vi "NM GlobalTest.vi"() -> ()   [LabVIEW 2010] (continued)
                      n358 = call "NITrapBlankChan.vi"("error in (no error)"=w832) -> ("error out"=w829:errorcluster)  [unwired: 9 in, 1 out]
                      n359 = call-poly <vilib>:"DAQmx Create Virtual Channel.vi"("task in"=w831, "high ticks"="high ticks", "low ticks"="low ticks", "counter"="DAQmx", "source of ticks"="source of ticks", "error in"=w829, "idle state"="idle state", "initial delay"="initial delay") -> ("task out"=w830:refnum<k21>, "error out"=w828:errorcluster)  [unwired: 6 in]
                      n360 = call "NITrapBlankChan.vi"("error in (no error)"=w828) -> ("error out"=w827:errorcluster)  [unwired: 9 in, 1 out]
                      n361 = call-poly <vilib>:"DAQmx Create Virtual Channel.vi"("task in"=w830, "high ticks"="high ticks", "low ticks"="low ticks", "counter"="DAQmx", "source of ticks"="source of ticks", "error in"=w827, "idle state"="idle state", "initial delay"="initial delay") -> ("task out"=w820:refnum<k21>, "error out"=w826:errorcluster)  [unwired: 6 in]
                      n362 = call "NITrapBlankChan.vi"("error in (no error)"=w826) -> ("message"=w818:string, "error out"=w819:errorcluster)  [unwired: 9 in]
                    }
                  }
                }
              }
            }
            frame "Composite In" {
              n363 = stacked-sequence {
                seq-local: [w846 _ _ _ _ _] -> [_ w867 _ _ _ _]
                seq-local: [w845 _ _ _ _ _] -> [_ w866 _ _ _ _]
                seq-local: [_ w865 _ _ _ _] -> [_ _ w881 _ _ _]
                seq-local: [_ w864 _ _ _ _] -> [_ _ w878 _ _ _]
                seq-local: [_ _ w880 _ _ _] -> [_ _ _ w908 _ _]
                seq-local: [_ _ w879 _ _ _] -> [_ _ _ w907 _ _]
                seq-local: [_ _ _ w906 _ _] -> [_ _ _ _ w916 _]
                seq-local: [_ _ _ w905 _ _] -> [_ _ _ _ w918 _]
                seq-local: [_ _ _ _ w916 _] -> [_ _ _ _ _ w927]
                seq-local: [_ _ _ _ w922 _] -> [_ _ _ _ _ w926]
                seq-local: ["ULx" _ _ _ _ _] -> [_ w857 _ _ _ _]
                seq-local: [_ w856 _ _ _ _] -> [_ _ w876 _ _ _]
                seq-local: [_ _ w875 _ _ _] -> [_ _ _ w893 _ _]
                seq-local: [_ _ _ w891 _ _] -> [_ _ _ _ w921 _]
                seq-local: [_ _ _ _ w919 _] -> [_ _ _ _ _ w924]
                tunnel: [_ _ _ _ _ w928] -> w837
                tunnel: [_ _ _ _ _ w929] -> w836
                tunnel: [_ _ _ _ _ w930] -> w835
                tunnel: [_ _ _ _ _ w923] -> w833
                frame #0 {
                  # "Composite Analog Input"
                  n364 = call-poly <vilib>:"ULx Create Virtual Channel.vi"("maximum value"="max", "minimum value"="min", "physical channels"="ULx") -> ("task out"=w855:refnum<k24>, "error out"=w853:errorcluster)  [unwired: 11 in]
                  n365 = call "TrapBlankChan.vi"("error in (no error)"=w853) -> ("error out"=w852:errorcluster)  [unwired: 9 in, 1 out]
                  n366 = call-poly <vilib>:"ULx Create Virtual Channel.vi"("task in"=w855, "maximum value"="max 9", "minimum value"="min 9", "physical channels"="physical channels 17", "error in"=w852) -> ("task out"=w854:refnum<k24>, "error out"=w851:errorcluster)  [unwired: 9 in]
                  n367 = call "TrapBlankChan.vi"("error in (no error)"=w851) -> ("error out"=w850:errorcluster)  [unwired: 9 in, 1 out]
                  n368 = call-poly <vilib>:"ULx Create Virtual Channel.vi"("task in"=w854, "maximum value"="max 12", "minimum value"="min 12", "physical channels"="physical channels 18", "error in"=w850) -> ("task out"=w846:refnum<k24>, "error out"=w849:errorcluster)  [unwired: 9 in]
                  n369 = call "TrapBlankChan.vi"("error in (no error)"=w849) -> ("error out"=w845:errorcluster)  [unwired: 9 in, 1 out]
                }
                frame #1 {
                  # "Composite Temperature Input"
                  n370 = call "StringJoiner.vi"("string 2"="ULx", "string 1"=w857) -> ("concatenated string"=w856:string)
                  n371 = call-poly <vilib>:"ULx Create Virtual Channel.vi"("task in"=w867, "physical channels"="ULx", "units"="units", "error in"=w866) -> ("task out"=w874:refnum<k24>, "error out"=w872:errorcluster)  [unwired: 10 in]
                  n372 = call "TrapBlankChan.vi"("error in (no error)"=w872) -> ("error out"=w871:errorcluster)  [unwired: 9 in, 1 out]
                  n373 = call-poly <vilib>:"ULx Create Virtual Channel.vi"("task in"=w874, "physical channels"="physical channels 20", "units"="units 7", "error in"=w871) -> ("task out"=w873:refnum<k24>, "error out"=w870:errorcluster)  [unwired: 10 in]
                  n374 = call "TrapBlankChan.vi"("error in (no error)"=w870) -> ("error out"=w869:errorcluster)  [unwired: 9 in, 1 out]
                  n375 = call-poly <vilib>:"ULx Create Virtual Channel.vi"("task in"=w873, "physical channels"="physical channels 21", "units"="units 12", "error in"=w869) -> ("task out"=w865:refnum<k24>, "error out"=w868:errorcluster)  [unwired: 10 in]
                  n376 = call "TrapBlankChan.vi"("error in (no error)"=w868) -> ("error out"=w864:errorcluster)  [unwired: 9 in, 1 out]
                }
                frame #2 {
                  # "Composite Digital Input"
                  n377 = call "StringJoiner.vi"("string 2"="ULx", "string 1"=w876) -> ("concatenated string"=w875:string)
                  n378 = call-poly <vilib>:"ULx Create Virtual Channel.vi"("task in"=w881, "ports"="ULx", "error in"=w878) -> ("task out"=w890:refnum<k24>, "error out"=w888:errorcluster)  [unwired: 11 in]
                  n379 = call "TrapBlankChan.vi"("error in (no error)"=w888) -> ("error out"=w887:errorcluster)  [unwired: 9 in, 1 out]
                  n380 = call-poly <vilib>:"ULx Create Virtual Channel.vi"("task in"=w890, "ports"="ports 2", "error in"=w887) -> ("task out"=w889:refnum<k24>, "error out"=w886:errorcluster)  [unwired: 11 in]
                  n381 = call "TrapBlankChan.vi"("error in (no error)"=w886) -> ("error out"=w885:errorcluster)  [unwired: 9 in, 1 out]
                  n382 = call-poly <vilib>:"ULx Create Virtual Channel.vi"("task in"=w889, "ports"="ports 3", "error in"=w885) -> ("task out"=w880:refnum<k24>, "error out"=w884:errorcluster)  [unwired: 11 in]
                  n383 = call "TrapBlankChan.vi"("error in (no error)"=w884) -> ("error out"=w879:errorcluster)  [unwired: 9 in, 1 out]
                }
                frame #3 {
                  # "Composite Counter Edge Input"
                  n384 = call "StringJoiner.vi"("string 2"="ULx", "string 1"=w893) -> ("concatenated string"=w891:string)
                  n385 = call-poly <vilib>:"ULx Create Virtual Channel.vi"("task in"=w908, "initial count"="initial count", "count direction"="direction", "edge"="edge", "counters"="ULx", "error in"=w907) -> ("task out"=w915:refnum<k24>, "error out"=w913:errorcluster)  [unwired: 8 in]
                  n386 = call "TrapBlankChan.vi"("error in (no error)"=w913) -> ("error out"=w912:errorcluster)  [unwired: 9 in, 1 out]
                  n387 = call-poly <vilib>:"ULx Create Virtual Channel.vi"("task in"=w915, "initial count"="initial count 5", "count direction"="direction 5", "edge"="edge 5", "counters"="counters 22", "error in"=w912) -> ("task out"=w914:refnum<k24>, "error out"=w911:errorcluster)  [unwired: 8 in]
                  n388 = call "TrapBlankChan.vi"("error in (no error)"=w911) -> ("error out"=w910:errorcluster)  [unwired: 9 in, 1 out]
                  n389 = call-poly <vilib>:"ULx Create Virtual Channel.vi"("task in"=w914, "initial count"="initial count 6", "count direction"="direction 6", "edge"="edge 6", "counters"="counters 23", "error in"=w910) -> ("task out"=w906:refnum<k24>, "error out"=w909:errorcluster)  [unwired: 8 in]
                  n390 = call "TrapBlankChan.vi"("error in (no error)"=w909) -> ("error out"=w905:errorcluster)  [unwired: 9 in, 1 out]
                }
                frame #4 {
                  # "Composite Encoder Input"
                  n391 = call "StringJoiner.vi"("string 2"="ULx", "string 1"=w921) -> ("concatenated string"=w919:string)
                  n392 = call "TrapBlankChan.vi"("error in (no error)"=w918) -> ("error out"=w917:errorcluster)  [unwired: 9 in, 1 out]
                  n393 = call "TrapBlankChan.vi"("error in (no error)"=w917) -> ("error out"=w922:errorcluster)  [unwired: 9 in, 1 out]
                }
                frame #5 {
                  n394 = call "StringJoiner.vi"("string 2"="ULx", "string 1"=w924) -> ("concatenated string"=w923:string)
                  n395 = call-poly <vilib>:"ULx Create Virtual Channel.vi"("task in"=w927, "maximum value"="max", "minimum value"="min", "physical channels"="ULx", "error in"=w926) -> ("task out"=w945:refnum<k24>, "error out"=w943:errorcluster)  [unwired: 9 in]
                  n396 = call "TrapBlankChan.vi"("error in (no error)"=w943) -> ("error out"=w942:errorcluster)  [unwired: 9 in, 1 out]
                  n397 = call-poly <vilib>:"ULx Create Virtual Channel.vi"("task in"=w945, "maximum value"="max 15", "minimum value"="min 15", "physical channels"="physical channels 29", "error in"=w942) -> ("task out"=w944:refnum<k24>, "error out"=w941:errorcluster)  [unwired: 9 in]
                  n398 = call "TrapBlankChan.vi"("error in (no error)"=w941) -> ("error out"=w940:errorcluster)  [unwired: 9 in, 1 out]
                  n399 = call-poly <vilib>:"ULx Create Virtual Channel.vi"("task in"=w944, "maximum value"="max 18", "minimum value"="min 18", "physical channels"="physical channels 30", "error in"=w940) -> ("task out"=w930:refnum<k24>, "error out"=w939:errorcluster)  [unwired: 9 in]
                  n400 = call "TrapBlankChan.vi"("error in (no error)"=w939) -> ("message"=w928:string, "error out"=w929:errorcluster)  [unwired: 9 in]
                }
              }
            }
            frame "Composite Out" {
              n401 = stacked-sequence {
                seq-local: [w961 _ _] -> [_ w977 _]
                seq-local: [w960 _ _] -> [_ w976 _]
                seq-local: [_ w975 _] -> [_ _ w992]
                seq-local: [_ w974 _] -> [_ _ w991]
                seq-local: ["ULx" _ _] -> [_ w971 _]
                seq-local: [_ w969 _] -> [_ _ w987]
                tunnel: [_ _ w990] -> w948
                tunnel: [_ _ w989] -> w950
                tunnel: [_ _ w988] -> w949
                tunnel: [_ _ w985] -> w946
                frame #0 {
                  # "Composite Analog Output"
                  n402 = call-poly <vilib>:"ULx Create Virtual Channel.vi"("maximum value"="max", "minimum value"="min", "physical channels"="ULx") -> ("task out"=w968:refnum<k24>, "error out"=w966:errorcluster)  [unwired: 11 in]
                  n403 = call "TrapBlankChan.vi"("error in (no error)"=w966) -> ("error out"=w965:errorcluster)  [unwired: 9 in, 1 out]
                  n404 = call-poly <vilib>:"ULx Create Virtual Channel.vi"("task in"=w968, "maximum value"="max 13", "minimum value"="min 13", "physical channels"="physical channels 23", "error in"=w965) -> ("task out"=w967:refnum<k24>, "error out"=w964:errorcluster)  [unwired: 9 in]
                  n405 = call "TrapBlankChan.vi"("error in (no error)"=w964) -> ("error out"=w963:errorcluster)  [unwired: 9 in, 1 out]
                  n406 = call-poly <vilib>:"ULx Create Virtual Channel.vi"("task in"=w967, "maximum value"="max 14", "minimum value"="min 14", "physical channels"="physical channels 24", "error in"=w963) -> ("task out"=w961:refnum<k24>, "error out"=w962:errorcluster)  [unwired: 9 in]
                  n407 = call "TrapBlankChan.vi"("error in (no error)"=w962) -> ("error out"=w960:errorcluster)  [unwired: 9 in, 1 out]
                }
                frame #1 {
                  # "Composite Digital Output"
                  n408 = call "StringJoiner.vi"("string 2"="ULx", "string 1"=w971) -> ("concatenated string"=w969:string)
                  n409 = call-poly <vilib>:"ULx Create Virtual Channel.vi"("task in"=w977, "ports"="ULx", "error in"=w976) -> ("task out"=w984:refnum<k24>, "error out"=w982:errorcluster)  [unwired: 11 in]
                  n410 = call "TrapBlankChan.vi"("error in (no error)"=w982) -> ("error out"=w981:errorcluster)  [unwired: 9 in, 1 out]
                  n411 = call-poly <vilib>:"ULx Create Virtual Channel.vi"("task in"=w984, "ports"="ports 5", "error in"=w981) -> ("task out"=w983:refnum<k24>, "error out"=w980:errorcluster)  [unwired: 11 in]
                  n412 = call "TrapBlankChan.vi"("error in (no error)"=w980) -> ("error out"=w979:errorcluster)  [unwired: 9 in, 1 out]
                  n413 = call-poly <vilib>:"ULx Create Virtual Channel.vi"("task in"=w983, "ports"="ports 6", "error in"=w979) -> ("task out"=w975:refnum<k24>, "error out"=w978:errorcluster)  [unwired: 11 in]
                  n414 = call "TrapBlankChan.vi"("error in (no error)"=w978) -> ("error out"=w974:errorcluster)  [unwired: 9 in, 1 out]
                }
                frame #2 {
                  # "Repeat Composite Analog Output"
                  n415 = call "StringJoiner.vi"("string 2"="ULx", "string 1"=w987) -> ("concatenated string"=w985:string)
                  n416 = call-poly <vilib>:"ULx Create Virtual Channel.vi"("task in"=w992, "maximum value"="max", "minimum value"="min", "physical channels"="ULx", "error in"=w991) -> ("task out"=w1007:refnum<k24>, "error out"=w1005:errorcluster)  [unwired: 9 in]
                  n417 = call "TrapBlankChan.vi"("error in (no error)"=w1005) -> ("error out"=w1004:errorcluster)  [unwired: 9 in, 1 out]
                  n418 = call-poly <vilib>:"ULx Create Virtual Channel.vi"("task in"=w1007, "maximum value"="max 16", "minimum value"="min 16", "physical channels"="physical channels 26", "error in"=w1004) -> ("task out"=w1006:refnum<k24>, "error out"=w1003:errorcluster)  [unwired: 9 in]
                  n419 = call "TrapBlankChan.vi"("error in (no error)"=w1003) -> ("error out"=w1002:errorcluster)  [unwired: 9 in, 1 out]
                  n420 = call-poly <vilib>:"ULx Create Virtual Channel.vi"("task in"=w1006, "maximum value"="max 17", "minimum value"="min 17", "physical channels"="physical channels 27", "error in"=w1002) -> ("task out"=w990:refnum<k24>, "error out"=w1001:errorcluster)  [unwired: 9 in]
                  n421 = call "TrapBlankChan.vi"("error in (no error)"=w1001) -> ("message"=w988:string, "error out"=w989:errorcluster)  [unwired: 9 in]
                }
              }
            }
          }
          n422 = local write "Active Channels"(w143) -> ()
          n423 = for {
            N: 5 -> [_]
            tunnel: w146 -> [w1009]
            tunnel: [FALSE] -> w145
            n424 = Wait Until Next ms Multiple(millisecond multiple=w1009) -> ()  [unwired: 1 out]
            "CreateChans" <- TRUE
          }
          n425 = case shown="No Error" w149 {
            selector: w149 -> [w1011 w1013]
            tunnel: [w1011 w1013] -> w152
            tunnel: w148 -> [_ w1012]
            frame No Error {
            }
            frame Error {
              "message 2" <- w1012
            }
          }
          n426 = local write "CreateChans"(w145) -> ()
        }
        frame 3 {
          # "Channel Info"
          n427 = Not Equal?(x="", y="Active Channels") -> (x != y?=w1014:bool)
          n428 = case shown="True" w1014 {
            tunnel: w1024 -> [w1033 w1041]
            tunnel: w1023 -> [w1032 w1040]
            tunnel: w1022 -> [w1031 w1039]
            tunnel: [w1033 w1038] -> w1021
            tunnel: [w1032 w1037] -> w1020
            tunnel: [w1031 w1036] -> w1019
            tunnel: w1018 -> [_ w1035]
            tunnel: "Active Channels" -> [_ w1034]
            frame False {
            }
            frame True {
              n429 = case shown="\"ULx\", Default" w1035 {
                tunnel: w1039 -> [w1045 w1053]
                tunnel: w1041 -> [w1047 w1052]
                tunnel: [w1047 w1051] -> w1038
                tunnel: [w1044 w1050] -> w1036
                tunnel: w1040 -> [w1043 w1049]
                tunnel: [w1042 w1049] -> w1037
                tunnel: w1034 -> [w1046 w1048]
                frame "ULx", Default {
                  n430 = call "SetActiveChans.vi"("error in (no error)"=w1045, "ActiveChannels"=w1046, "task in"=w1043) -> ("error out"=w1044:errorcluster, "task out"=w1042:refnum<k24>)
                }
                frame "DAQmx" {
                  n431 = property class="DAQmx Channel"(reference=w1052, error in=w1053, "ActiveChans"=w1048) -> (reference out=w1051:refnum<k21>, error out=w1050:errorcluster)
                }
              }
            }
          }
          n432 = call "DAQmxTaskInfo.vi"("task in"=w1021) -> ("ChanType"=→"ChanType":i32, "Name"=→"Name":refnum<k21>)
          n433 = call "ULxTaskInfo.vi"("task in"=w1020) -> ("NumberOfChannels"=→"NumberOfChannels":u32, "Task"=→"Task":i32, "ToString"=→"ToString":string)
          n434 = local read "SelLib"() -> (w1025:enum32{"ULx", "DAQmx"})
          n435 = case shown="\"ULx\", Default" w1025 {
            tunnel: w1021 -> [_ w1058]
            tunnel: w1020 -> [w1056 _]
            tunnel: [w1054 w1057] -> w1026
            frame "ULx", Default {
              n436 = call "ULxTaskInfo.vi"("task in"=w1056) -> ("Task"=w1055:i32)  [unwired: 2 out]
              n437 = Number To Hexadecimal String(2:w1055) -> (0:w1054:string)  [unwired: 1 in]
            }
            frame "DAQmx" {
              n438 = call "DAQmxTaskInfo.vi"("task in"=w1058) -> ("Name"=w1057:refnum<k21>)  [unwired: 1 out]
            }
          }
          "String" <- w1026
        }
        frame 4 {
          # "TIMING"
          n439 = for {
            N: 5 -> [_]
            tunnel: w1061 -> [w1073]
            tunnel: [FALSE] -> w1060
            n440 = Wait Until Next ms Multiple(millisecond multiple=w1073) -> ()  [unwired: 1 out]
            "Timing" <- TRUE
          }
          n441 = local write "Timing"(w1060) -> ()
          n442 = case shown="\"Clock\", Default" "Tab Control" {
            tunnel: w1067 -> [w1081 w1107 w1128]
            tunnel: w1066 -> [w1080 w1106 w1127]
            tunnel: [w1079 w1105 w1126] -> w1064
            tunnel: [w1078 w1104 w1125] -> w1063
            tunnel: w1069 -> [w1077 w1103 w1124]
            tunnel: w1068 -> [w1076 w1102 w1123]
            tunnel: [w1075 w1101 w1122] -> w1065
            frame "Clock", Default {
              n443 = case shown="\"DAQmx\"" w1077 {
                tunnel: w1081 -> [w1090 w1091]
                tunnel: w1080 -> [w1089 w1100]
                tunnel: [w1088 w1091] -> w1079
                tunnel: [w1087 w1099] -> w1078
                tunnel: w1076 -> [w1082 w1098]
                tunnel: [w1082 w1097] -> w1075
                frame "ULx", Default {
                  n444 = call-poly <vilib>:"ULx Timing.vi"("task in"=w1090, "sample mode"="sample mode", "samples per channel"="samples per", "rate"="rate", "clock source"="clock source", "error in"=w1089) -> ("task out"=w1088:refnum<k24>, "error out"=w1087:errorcluster)  [unwired: 8 in]
                }
                frame "DAQmx" {
                  n445 = call-poly <vilib>:"DAQmx Timing.vi"("task/channels in"=w1098, "sample mode"="sample mode", "samples per channel"="samples per", "rate"="mxRate", "source"="source", "active edge"="active edge", "error in"=w1100) -> ("task out"=w1097:refnum<k21>, "error out"=w1099:errorcluster)  [unwired: 7 in]
                }
              }
            }
            frame "Waveform" {
              n446 = case shown="\"ULx\", Default" w1103 {
                tunnel: w1107 -> [w1114 w1115]
                tunnel: w1106 -> [w1113 w1121]
                tunnel: [w1112 w1115] -> w1105
                tunnel: [w1111 w1120] -> w1104
                tunnel: w1102 -> [w1108 w1119]
                tunnel: [w1108 w1118] -> w1101
                frame "ULx", Default {
                  n447 = call-poly <vilib>:"ULx Timing.vi"("task in"=w1114, "sample mode"="sample mode 3", "waveform"="waveform", "error in"=w1113) -> ("task out"=w1112:refnum<k24>, "error out"=w1111:errorcluster)  [unwired: 10 in]
                }
                frame "DAQmx" {
                  n448 = call-poly <vilib>:"DAQmx Timing.vi"("task/channels in"=w1119, "sample mode"="sample mode 2", "waveform"="waveform 2", "error in"=w1121) -> ("task out"=w1118:refnum<k21>, "error out"=w1120:errorcluster)  [unwired: 10 in]
                }
              }
            }
            frame "Implicit" {
              n449 = case shown="\"ULx\", Default" w1124 {
                tunnel: w1128 -> [w1135 w1136]
                tunnel: w1127 -> [w1134 w1142]
                tunnel: [w1133 w1136] -> w1126
                tunnel: [w1132 w1141] -> w1125
                tunnel: w1123 -> [w1131 w1140]
                tunnel: [w1131 w1139] -> w1122
                frame "ULx", Default {
                  n450 = call-poly <vilib>:"ULx Timing.vi"("task in"=w1135, "sample mode"="sample mode", "samples per channel"="samples per channel", "error in"=w1134) -> ("task out"=w1133:refnum<k24>, "error out"=w1132:errorcluster)  [unwired: 10 in]
                }
                frame "DAQmx" {
                  n451 = call-poly <vilib>:"DAQmx Timing.vi"("task/channels in"=w1140, "sample mode"="sample mode", "samples per channel"="samples per channel", "error in"=w1142) -> ("task out"=w1139:refnum<k21>, "error out"=w1141:errorcluster)  [unwired: 10 in]
                }
              }
            }
          }
          n452 = case shown="True" "Once" {
            frame False {
            }
            frame True {
              n453 = local write "Timing"(FALSE ("Timing")) -> ()
            }
          }
        }
        frame 5 {
          # "TRIGGERING"
          n454 = for {
            N: 5 -> [_]
            tunnel: w1145 -> [w1161]
            tunnel: [FALSE] -> w1144
            n455 = Wait Until Next ms Multiple(millisecond multiple=w1161) -> ()  [unwired: 1 out]
            "Trigger" <- TRUE
          }
          n456 = case shown="\"Basic\", Default" "TrigType" {
            tunnel: [w1169 w1241 w1292 w1348] -> w1156
            tunnel: [w1170 w1240 w1293 w1349] -> w1157
            tunnel: "BasicType" -> [w1168 _ _ _]
            tunnel: "GatedType" -> [_ w1239 _ _]
            tunnel: "StartType" -> [_ _ w1294 _]
            tunnel: "StopType" -> [_ _ _ w1350]
            tunnel: [w1167 w1238 w1290 w1344] -> w1158
            tunnel: w1150 -> [w1165 w1236 w1289 w1347]
            tunnel: w1149 -> [w1164 w1235 w1288 w1346]
            tunnel: w1148 -> [w1166 w1237 w1291 w1345]
            tunnel: w1147 -> [w1163 w1234 _ _]
            frame "Basic", Default {
              n457 = case shown="\"DPtrn\"" w1168 {
                tunnel: [w1177 w1194 w1213 w1219 w1231] -> w1170
                tunnel: [w1176 w1193 w1214 w1218 w1232] -> w1169
                tunnel: [w1175 w1192 w1215 w1225 w1233] -> w1167
                tunnel: w1166 -> [w1174 w1191 w1215 w1225 w1233]
                tunnel: w1165 -> [w1173 w1190 w1209 w1217 w1227]
                tunnel: w1164 -> [w1172 w1189 w1210 w1216 w1226]
                tunnel: w1163 -> [w1171 w1188 _ _ _]
                frame "None", Default {
                  n458 = case shown="\"ULx\", Default" w1171 {
                    tunnel: [w1181 w1184] -> w1177
                    tunnel: [w1180 w1187] -> w1176
                    tunnel: [w1182 w1186] -> w1175
                    tunnel: w1174 -> [w1182 w1185]
                    tunnel: w1173 -> [w1179 w1184]
                    tunnel: w1172 -> [w1178 w1183]
                    frame "ULx", Default {
                      n459 = call-poly <vilib>:"ULx Trigger.vi"("task in"=w1179, "error in"=w1178) -> ("task out"=w1181:refnum<k24>, "error out"=w1180:errorcluster)  [unwired: 16 in]
                    }
                    frame "DAQmx" {
                      n460 = call-poly <vilib>:"DAQmx Trigger.vi"("task/channels in"=w1185, "error in"=w1183) -> ("task out"=w1186:refnum<k21>, "error out"=w1187:errorcluster)  [unwired: 12 in]
                    }
                  }
                }
                frame "DEdge" {
                  n461 = case shown="\"ULx\", Default" w1188 {
                    tunnel: [w1198 w1203] -> w1194
                    tunnel: [w1199 w1208] -> w1193
                    tunnel: [w1201 w1207] -> w1192
                    tunnel: w1191 -> [w1201 w1204]
                    tunnel: w1190 -> [w1195 w1203]
                    tunnel: w1189 -> [w1196 w1202]
                    frame "ULx", Default {
                      n462 = call-poly <vilib>:"ULx Trigger.vi"("task in"=w1195, "edge"="ULx edge", "error in"=w1196, "pretrigger samples per channel"="pretrigger samples per channel") -> ("task out"=w1198:refnum<k24>, "error out"=w1199:errorcluster)  [unwired: 14 in]
                    }
                    frame "DAQmx" {
                      n463 = call-poly <vilib>:"DAQmx Trigger.vi"("task/channels in"=w1204, "source"="DAQmx source", "edge"="DAQmx edge", "error in"=w1202) -> ("task out"=w1207:refnum<k21>, "error out"=w1208:errorcluster)  [unwired: 10 in]
                    }
                  }
                }
                frame "DLevel" {
                  n464 = call-poly <vilib>:"ULx Trigger.vi"("task in"=w1209, "level"="level", "error in"=w1210, "pretrigger samples per channel"="pretrigger samples per channel") -> ("task out"=w1213:refnum<k24>, "error out"=w1214:errorcluster)  [unwired: 14 in]
                }
                frame "DPtrn" {
                  n465 = call-poly <vilib>:"ULx Trigger.vi"("task in"=w1217, "trigger channel"="trig chan", "trigger sensitivity"="sensitivity", "pattern"="pattern", "mask"="mask", "error in"=w1216, "pretrigger samples per channel"="Pretrig Samps") -> ("task out"=w1219:refnum<k24>, "error out"=w1218:errorcluster)  [unwired: 11 in]
                }
                frame "AEdge" {
                  n466 = call-poly <vilib>:"ULx Trigger.vi"("task in"=w1227, "slope"="slope", "level"="level", "error in"=w1226, "pretrigger samples per channel"="pretrigger samples per channel") -> ("task out"=w1231:refnum<k24>, "error out"=w1232:errorcluster)  [unwired: 13 in]
                }
              }
            }
            frame "Gated" {
              n467 = case shown="\"None\", Default" w1239 {
                tunnel: [w1247 w1263 w1270 w1278 w1286] -> w1241
                tunnel: [w1248 w1262 w1269 w1277 w1285] -> w1240
                tunnel: [w1246 w1264 w1271 w1279 w1287] -> w1238
                tunnel: w1237 -> [w1245 w1264 w1271 w1279 w1287]
                tunnel: w1236 -> [w1244 w1259 w1265 w1272 w1280]
                tunnel: w1235 -> [w1243 w1260 w1266 w1273 w1281]
                tunnel: w1234 -> [w1242 _ _ _ _]
                frame "None", Default {
                  n468 = case shown="\"ULx\", Default" w1242 {
                    tunnel: [w1252 w1255] -> w1248
                    tunnel: [w1251 w1258] -> w1247
                    tunnel: [w1253 w1257] -> w1246
                    tunnel: w1245 -> [w1253 w1256]
                    tunnel: w1244 -> [w1249 w1255]
                    tunnel: w1243 -> [w1250 w1254]
                    frame "ULx", Default {
                      n469 = call-poly <vilib>:"ULx Trigger.vi"("task in"=w1249, "error in"=w1250) -> ("task out"=w1252:refnum<k24>, "error out"=w1251:errorcluster)  [unwired: 16 in]
                    }
                    frame "DAQmx" {
                      n470 = call-poly <vilib>:"DAQmx Trigger.vi"("task/channels in"=w1256, "error in"=w1254) -> ("task out"=w1257:refnum<k21>, "error out"=w1258:errorcluster)  [unwired: 12 in]
                    }
                  }
                }
                frame "DLevel" {
                  n471 = call-poly <vilib>:"ULx Trigger.vi"("task in"=w1259, "level"="Level 3", "error in"=w1260) -> ("task out"=w1262:refnum<k24>, "error out"=w1263:errorcluster)  [unwired: 15 in]
                }
                frame "ALevel" {
                  n472 = call-poly <vilib>:"ULx Trigger.vi"("task in"=w1265, "position"="position", "level"="level", "error in"=w1266) -> ("task out"=w1269:refnum<k24>, "error out"=w1270:errorcluster)  [unwired: 14 in]
                }
                frame "AWindow" {
                  n473 = call-poly <vilib>:"ULx Trigger.vi"("task in"=w1272, "When"="When", "window bottom"="bottom", "window top"="top", "error in"=w1273) -> ("task out"=w1277:refnum<k24>, "error out"=w1278:errorcluster)  [unwired: 13 in]
                }
                frame "AHyst" {
                  n474 = call-poly <vilib>:"ULx Trigger.vi"("task in"=w1280, "hysteresis"="hyst", "low threshold"="low", "high threshold"="high", "error in"=w1281) -> ("task out"=w1285:refnum<k24>, "error out"=w1286:errorcluster)  [unwired: 13 in]
                }
              }
            }
            frame "Start" {
              n475 = case shown="\"None\", Default" w1294 {
                tunnel: [w1298 w1303 w1311 w1321 w1331 w1341] -> w1293
                tunnel: [w1295 w1304 w1312 w1322 w1332 w1342] -> w1292
                tunnel: [w1299 w1305 w1313 w1323 w1333 w1343] -> w1290
                tunnel: w1291 -> [w1299 w1305 w1313 w1323 w1333 w1343]
                tunnel: w1289 -> [w1297 w1301 w1306 w1314 w1324 w1334]
                tunnel: w1288 -> [w1296 w1302 w1307 w1315 w1325 w1335]
                frame "None", Default {
                  n476 = call-poly <vilib>:"ULx Trigger.vi"("task in"=w1297, "error in"=w1296) -> ("task out"=w1298:refnum<k24>, "error out"=w1295:errorcluster)  [unwired: 16 in]
                }
                frame "ExtTTL" {
                  n477 = call-poly <vilib>:"ULx Trigger.vi"("task in"=w1301, "trigger sensitivity"="trigger sensitivity", "error in"=w1302) -> ("task out"=w1303:refnum<k24>, "error out"=w1304:errorcluster)  [unwired: 15 in]
                }
                frame "AHdwr" {
                  n478 = call-poly <vilib>:"ULx Trigger.vi"("task in"=w1306, "trigger sensitivity"="sensitivity", "level"="Level", "variance"="variance", "error in"=w1307) -> ("task out"=w1311:refnum<k24>, "error out"=w1312:errorcluster)  [unwired: 13 in]
                }
                frame "ASftwr" {
                  n479 = call-poly <vilib>:"ULx Trigger.vi"("task in"=w1314, "trigger channel"="trigger channel", "trigger sensitivity"="sensitivity", "level"="Level", "variance"="variance", "error in"=w1315, "pretrigger samples per channel"="pretrigger samples") -> ("task out"=w1321:refnum<k24>, "error out"=w1322:errorcluster)  [unwired: 11 in]
                }
                frame "DPtrn" {
                  n480 = call-poly <vilib>:"ULx Trigger.vi"("task in"=w1324, "trigger channel"="trigger channel", "trigger sensitivity"="trigger sensitivity", "pattern"="level", "variance"="variance", "error in"=w1325, "pretrigger samples per channel"="pretrigger samples") -> ("task out"=w1331:refnum<k24>, "error out"=w1332:errorcluster)  [unwired: 11 in]
                }
                frame "Ctr" {
                  n481 = call-poly <vilib>:"ULx Trigger.vi"("task in"=w1334, "trigger channel"="trigger channel", "trigger sensitivity"="trigger sensitivity", "count"="level", "variance"="variance", "error in"=w1335, "pretrigger samples per channel"="pretrigger samples") -> ("task out"=w1341:refnum<k24>, "error out"=w1342:errorcluster)  [unwired: 11 in]
                }
              }
            }
            frame "Stop" {
              n482 = case shown="\"None\", Default" w1350 {
                tunnel: [w1351 w1362 w1371 w1380] -> w1349
                tunnel: [w1353 w1363 w1372 w1381] -> w1348
                tunnel: w1347 -> [w1352 w1357 w1365 w1374]
                tunnel: w1346 -> [w1354 w1356 w1366 w1375]
                tunnel: w1345 -> [w1355 w1364 w1373 w1382]
                tunnel: [w1355 w1364 w1373 w1382] -> w1344
                frame "None", Default {
                  n483 = call-poly <vilib>:"ULx Trigger.vi"("task in"=w1352, "error in"=w1354) -> ("task out"=w1351:refnum<k24>, "error out"=w1353:errorcluster)  [unwired: 16 in]
                }
                frame "ASftwr" {
                  n484 = call-poly <vilib>:"ULx Trigger.vi"("task in"=w1357, "trigger channel"="trigger channel", "trigger sensitivity"="trigger sensitivity", "level"="level", "variance"="variance", "error in"=w1356) -> ("task out"=w1362:refnum<k24>, "error out"=w1363:errorcluster)  [unwired: 12 in]
                }
                frame "DPtrn" {
                  n485 = call-poly <vilib>:"ULx Trigger.vi"("task in"=w1365, "trigger channel"="trigger channel", "trigger sensitivity"="trigger sensitivity", "pattern"="level", "variance"="variance", "error in"=w1366) -> ("task out"=w1371:refnum<k24>, "error out"=w1372:errorcluster)  [unwired: 12 in]
                }
                frame "Ctr" {
                  n486 = call-poly <vilib>:"ULx Trigger.vi"("task in"=w1374, "trigger channel"="trigger channel", "trigger sensitivity"="trigger sensitivity", "count"="level", "variance"="variance", "error in"=w1375) -> ("task out"=w1380:refnum<k24>, "error out"=w1381:errorcluster)  [unwired: 12 in]
                }
              }
            }
          }
          n487 = local write "Trigger"(w1144) -> ()
          n488 = case shown="True" "Once" {
            frame False {
            }
            frame True {
              n489 = local write "Trig"(FALSE ("Trig")) -> ()
            }
          }
        }
        frame 6 {
          # "START"
          n490 = for {
            N: 5 -> [_]
            tunnel: w1391 -> [w1401]
            tunnel: w1390 -> [w1400]
            tunnel: [FALSE] -> w1389
            n491 = case shown="1" w1400 {
              tunnel: TRUE -> [w1402 w1403]
              frame 0, Default {
                "Start" <- w1402
              }
              frame 1 {
                "Start 2" <- w1403
              }
            }
            n492 = Wait Until Next ms Multiple(millisecond multiple=w1401) -> ()  [unwired: 1 out]
          }
          n493 = case shown="\"DAQmx\"" w1386 {
            tunnel: w1394 -> [w1408 w1409]
            tunnel: [w1407 w1409] -> w1384
            tunnel: [w1406 w1412] -> w1383
            tunnel: w1393 -> [w1405 w1413]
            tunnel: w1395 -> [w1404 w1411]
            tunnel: [w1404 w1410] -> w1385
            frame "ULx", Default {
              n494 = call <vilib>:"ULx Start Task.vi"("task in"=w1408, "error in"=w1405) -> ("task out"=w1407:refnum<k24>, "error out"=w1406:errorcluster)  [unwired: 12 in]
            }
            frame "DAQmx" {
              n495 = call <vilib>:"DAQmx Start Task.vi"("task/channels in"=w1411, "error in"=w1413) -> ("task out"=w1410:refnum<k21>, "error out"=w1412:errorcluster)  [unwired: 12 in]
            }
          }
          n496 = local write "Start"(w1389) -> ()
          n497 = local write "Start 2"(w1389) -> ()
          n498 = case shown="True" "Once" {
            frame False {
            }
            frame True {
              n499 = local write "Start"(FALSE ("Start")) -> ()
            }
          }
          n500 = case shown="True" "Once" {
            frame False {
            }
            frame True {
              n501 = local write "Start"(FALSE ("Start")) -> ()
            }
          }
        }
        frame 7 {
          # "WRITE"
          n502 = property on="samples" class="DigNum (strict)"("Maximum"="samps") -> ()  [unwired: 2 in, 2 out]
          n503 = call "Complicated Function Generator.vi"("frequency"="freq", "signal type"="sig type", "offset"="offset", "amplitude"="ampl", "samples"="samps", "bufsize"="samps", "Chans"="Chans") -> ("Wave out"=w1424:waveform(dbl), "WfmArray"=w1422:waveform(dbl)[], "DblArray"=w1423:dbl[][], "DBL Out"=w1419:dbl[])  [unwired: 3 in, 2 out]
          n504 = case shown="False" "Mod Array" {
            tunnel: "Chans" -> [_ w1443]
            tunnel: w1419 -> [w1437 w1442]
            tunnel: [w1437 w1438] -> w1418
            frame False {
            }
            frame True {
              n505 = call "Complicated Function Generator.vi"("frequency"="freq", "signal type"="signal type", "amplitude"="atude", "samples"="samples", "bufsize"="samples", "Chans"=w1443) -> ("DBL Out"=w1445:dbl[])  [unwired: 4 in, 5 out]
              n506 = Replace Array Subset(array=w1442, new element=w1445, index="index") -> (w1438:dbl[])
            }
          }
          n507 = stacked-sequence {
            tunnel: w1435 -> [_ w1470]
            tunnel: w1434 -> [_ w1461]
            tunnel: w1433 -> [_ w1460]
            tunnel: w1432 -> [_ w1459]
            tunnel: [_ w1466] -> w1431
            tunnel: [_ w1465] -> w1430
            tunnel: [_ w1464] -> w1429
            tunnel: w1428 -> [w1447 _]
            tunnel: [_ FALSE] -> w1427
            tunnel: w1418 -> [_ w1454]
            tunnel: w1424 -> [_ w1458]
            tunnel: w1423 -> [_ w1457]
            tunnel: w1422 -> [_ w1456]
            tunnel: "samps" -> [_ w1455]
            tunnel: "sig type" -> [_ w1453]
            tunnel: "Chans" -> [_ w1451]
            frame #0 {
              n508 = for {
                N: 5 -> [_]
                tunnel: w1447 -> [w1450]
                n509 = Wait Until Next ms Multiple(millisecond multiple=w1450) -> ()  [unwired: 1 out]
                "Write" <- TRUE ("Write")
              }
            }
            frame #1 {
              n510 = case shown="\"Counter\"" "TaskType 2" {
                tunnel: w1459 -> [w1493 w1804 w2420 w2647]
                tunnel: w1460 -> [w1492 w1803 w2421 w2648]
                tunnel: w1461 -> [w1491 w1802 w2422 w2649]
                tunnel: w1470 -> [w1489 w1801 w2419 w2646]
                tunnel: [w1486 w1797 w2415 w2645] -> w1464
                tunnel: [w1488 w1799 w2417 w2644] -> w1466
                tunnel: [w1487 w1798 w2416 w2643] -> w1465
                tunnel: "AutoStart" -> [w1485 w1796 w2414 w2642]
                tunnel: [w1484 w1794 w2412 w2640] -> w1468
                tunnel: "TO" -> [w1483 w1795 w2413 w2641]
                tunnel: w1454 -> [w1482 w1793 _ w2636]
                tunnel: w1458 -> [w1481 _ _ _]
                tunnel: w1457 -> [w1480 _ _ w2639]
                tunnel: w1456 -> [w1479 _ _ w2638]
                tunnel: w1455 -> [_ w1792 _ w2637]
                tunnel: w1451 -> [_ _ _ w2634]
                frame "Analog", Default {
                  n511 = case shown="\"sCnS1D\"" "AWrite" {
                    tunnel: [w1503 w1533 w1559 w1586 w1615 w1644 w1673 w1705 w1730 w1754 w1776] -> w1486
                    tunnel: [w1504 w1532 w1558 w1587 w1616 w1645 w1674 w1706 w1731 w1753 w1775] -> w1487
                    tunnel: w1492 -> [w1501 w1531 w1561 w1589 w1619 w1648 w1677 w1703 w1734 w1756 w1778]
                    tunnel: w1491 -> [w1502 w1529 w1562 w1591 w1620 w1649 w1678 w1704 w1735 w1755 w1777]
                    tunnel: w1493 -> [w1500 w1530 w1560 w1590 w1618 w1647 w1676 w1702 w1733 w1757 w1779]
                    tunnel: [w1499 w1528 w1557 w1588 w1617 w1646 w1675 w1707 w1732 w1752 w1774] -> w1488
                    tunnel: w1489 -> [w1497 w1526 w1556 w1585 w1613 w1642 w1672 w1701 w1729 w1751 w1773]
                    tunnel: w1485 -> [w1496 w1525 w1555 w1584 w1611 w1640 w1671 w1700 w1728 w1750 w1772]
                    tunnel: [w1494 w1523 w1554 w1583 w1610 w1639 w1670 w1699 w1727 w1748 w1770] -> w1484
                    tunnel: w1483 -> [w1495 w1524 w1553 w1582 w1612 w1641 w1669 w1698 w1726 w1749 w1771]
                    tunnel: w1482 -> [_ _ w1552 _ _ _ _ _ _ _ _]
                    tunnel: w1481 -> [_ _ _ w1581 _ _ _ _ _ _ _]
                    tunnel: w1480 -> [_ _ _ _ _ _ w1668 _ _ _ _]
                    tunnel: w1479 -> [_ _ _ _ _ _ _ w1697 _ _ _]
                    frame "sCsSDbl", Default {
                      n512 = case shown="\"ULx\", Default" w1497 {
                        tunnel: [w1509 w1514] -> w1504
                        tunnel: [w1510 w1518] -> w1503
                        tunnel: w1502 -> [w1505 w1521]
                        tunnel: w1501 -> [w1512 w1514]
                        tunnel: w1500 -> [w1511 w1522]
                        tunnel: [w1505 w1519] -> w1499
                        tunnel: "data 2" -> [w1513 w1520]
                        tunnel: w1496 -> [w1508 w1517]
                        tunnel: w1495 -> [w1507 w1515]
                        tunnel: [w1506 w1516] -> w1494
                        frame "ULx", Default {
                          n513 = call-poly <vilib>:"ULx Write.vi"("task in"=w1512, "auto start"=w1508, "data"=w1513, "timeout"=w1507, "error in"=w1511) -> ("task out"=w1509:refnum<k24>, "number of samples written per channel"=w1506:u32, "error out"=w1510:errorcluster)  [unwired: 8 in]
                        }
                        frame "DAQmx" {
                          n514 = call-poly <vilib>:"DAQmx Write.vi"("task/channels in"=w1521, "auto start"=w1517, "data"=w1520, "timeout"=w1515, "error in"=w1522) -> ("task out"=w1519:refnum<k21>, "number of samples written per channel"=w1516:u32, "error out"=w1518:errorcluster)  [unwired: 8 in]
                        }
                      }
                    }
                    frame "sCsSWfm" {
                      n515 = case shown="\"ULx\", Default" w1526 {
                        tunnel: [w1539 w1548] -> w1533
                        tunnel: [w1540 w1543] -> w1532
                        tunnel: w1531 -> [w1542 w1543]
                        tunnel: w1530 -> [w1541 w1550]
                        tunnel: w1529 -> [w1534 w1551]
                        tunnel: [w1534 w1549] -> w1528
                        tunnel: "data" -> [w1538 w1547]
                        tunnel: w1525 -> [w1537 w1546]
                        tunnel: w1524 -> [w1536 w1544]
                        tunnel: [w1535 w1545] -> w1523
                        frame "ULx", Default {
                          n516 = call-poly <vilib>:"ULx Write.vi"("task in"=w1542, "auto start"=w1537, "data"=w1538, "timeout"=w1536, "error in"=w1541) -> ("task out"=w1540:refnum<k24>, "number of samples written per channel"=w1535:u32, "error out"=w1539:errorcluster)  [unwired: 8 in]
                        }
                        frame "DAQmx" {
                          n517 = call-poly <vilib>:"DAQmx Write.vi"("task/channels in"=w1551, "auto start"=w1546, "data"=w1547, "timeout"=w1544, "error in"=w1550) -> ("task out"=w1549:refnum<k21>, "number of samples written per channel"=w1545:u32, "error out"=w1548:errorcluster)  [unwired: 8 in]
                        }
                      }
                    }
                    frame "sCnS1D" {
                      n518 = case shown="\"DAQmx\"" w1556 {
                        tunnel: [w1568 w1577] -> w1559
                        tunnel: w1562 -> [w1563 w1580]
                        tunnel: w1561 -> [w1571 w1573]
                        tunnel: w1560 -> [w1570 w1579]
                        tunnel: [w1569 w1573] -> w1558
                        tunnel: [w1563 w1578] -> w1557
                        tunnel: w1552 -> [w1567 w1576]
                        tunnel: w1555 -> [w1566 w1572]
                        tunnel: [w1565 w1575] -> w1554
                        tunnel: w1553 -> [w1564 w1574]
                        frame "ULx", Default {
                          n519 = call-poly <vilib>:"ULx Write.vi"("task in"=w1571, "auto start"=w1566, "data"=w1567, "timeout"=w1564, "error in"=w1570) -> ("task out"=w1569:refnum<k24>, "number of samples written per channel"=w1565:u32, "error out"=w1568:errorcluster)  [unwired: 8 in]
                        }
                        frame "DAQmx" {
                          n520 = call-poly <vilib>:"DAQmx Write.vi"("task/channels in"=w1580, "auto start"=w1572, "data"=w1576, "timeout"=w1574, "error in"=w1579) -> ("task out"=w1578:refnum<k21>, "number of samples written per channel"=w1575:u32, "error out"=w1577:errorcluster)  [unwired: 8 in]
                        }
                      }
                      "data 3" <- w1552
                      "DBL Out" <- w1552
                    }
                    frame "sCnSWfm" {
                      n521 = case shown="\"ULx\", Default" w1585 {
                        tunnel: [w1598 w1601] -> w1587
                        tunnel: [w1597 w1606] -> w1586
                        tunnel: w1591 -> [w1592 w1608]
                        tunnel: w1589 -> [w1600 w1601]
                        tunnel: w1590 -> [w1599 w1609]
                        tunnel: [w1592 w1607] -> w1588
                        tunnel: w1581 -> [w1596 w1605]
                        tunnel: w1584 -> [w1595 w1603]
                        tunnel: [w1594 w1602] -> w1583
                        tunnel: w1582 -> [w1593 w1604]
                        frame "ULx", Default {
                          n522 = call-poly <vilib>:"ULx Write.vi"("task in"=w1600, "auto start"=w1595, "data"=w1596, "timeout"=w1593, "error in"=w1599) -> ("task out"=w1598:refnum<k24>, "number of samples written per channel"=w1594:u32, "error out"=w1597:errorcluster)  [unwired: 8 in]
                        }
                        frame "DAQmx" {
                          n523 = call-poly <vilib>:"DAQmx Write.vi"("task/channels in"=w1608, "auto start"=w1603, "data"=w1605, "timeout"=w1604, "error in"=w1609) -> ("task out"=w1607:refnum<k21>, "number of samples written per channel"=w1602:u32, "error out"=w1606:errorcluster)  [unwired: 8 in]
                        }
                      }
                      "data 4" <- w1581
                    }
                    frame "nCsSDbl" {
                      n524 = case shown="\"ULx\", Default" w1613 {
                        tunnel: [w1627 w1630] -> w1616
                        tunnel: [w1626 w1635] -> w1615
                        tunnel: w1620 -> [w1621 w1637]
                        tunnel: w1619 -> [w1629 w1630]
                        tunnel: w1618 -> [w1628 w1638]
                        tunnel: [w1621 w1636] -> w1617
                        tunnel: "data 5" -> [w1625 w1634]
                        tunnel: w1612 -> [w1624 w1632]
                        tunnel: w1611 -> [w1623 w1631]
                        tunnel: [w1622 w1633] -> w1610
                        frame "ULx", Default {
                          n525 = call-poly <vilib>:"ULx Write.vi"("task in"=w1629, "auto start"=w1623, "data"=w1625, "timeout"=w1624, "error in"=w1628) -> ("task out"=w1627:refnum<k24>, "number of samples written per channel"=w1622:u32, "error out"=w1626:errorcluster)  [unwired: 8 in]
                        }
                        frame "DAQmx" {
                          n526 = call-poly <vilib>:"DAQmx Write.vi"("task/channels in"=w1637, "auto start"=w1631, "data"=w1634, "timeout"=w1632, "error in"=w1638) -> ("task out"=w1636:refnum<k21>, "number of samples written per channel"=w1633:u32, "error out"=w1635:errorcluster)  [unwired: 8 in]
                        }
                      }
                    }
                    frame "nCsSWfm" {
                      n527 = case shown="\"ULx\", Default" w1642 {
                        tunnel: [w1656 w1659] -> w1645
                        tunnel: [w1655 w1664] -> w1644
                        tunnel: w1649 -> [w1650 w1666]
                        tunnel: w1648 -> [w1658 w1659]
                        tunnel: w1647 -> [w1657 w1667]
                        tunnel: [w1650 w1665] -> w1646
                        tunnel: "data 6" -> [w1654 w1663]
                        tunnel: w1641 -> [w1653 w1660]
                        tunnel: w1640 -> [w1652 w1661]
                        tunnel: [w1651 w1662] -> w1639
                        frame "ULx", Default {
                          n528 = call-poly <vilib>:"ULx Write.vi"("task in"=w1658, "auto start"=w1652, "data"=w1654, "timeout"=w1653, "error in"=w1657) -> ("task out"=w1656:refnum<k24>, "number of samples written per channel"=w1651:u32, "error out"=w1655:errorcluster)  [unwired: 8 in]
                        }
                        frame "DAQmx" {
                          n529 = call-poly <vilib>:"DAQmx Write.vi"("task/channels in"=w1666, "auto start"=w1661, "data"=w1663, "timeout"=w1660, "error in"=w1667) -> ("task out"=w1665:refnum<k21>, "number of samples written per channel"=w1662:u32, "error out"=w1664:errorcluster)  [unwired: 8 in]
                        }
                      }
                    }
                    frame "nCnS2D" {
                      n530 = case shown="\"ULx\", Default" w1672 {
                        tunnel: [w1685 w1688] -> w1674
                        tunnel: [w1684 w1693] -> w1673
                        tunnel: w1678 -> [w1679 w1695]
                        tunnel: w1677 -> [w1687 w1688]
                        tunnel: w1676 -> [w1686 w1696]
                        tunnel: [w1679 w1694] -> w1675
                        tunnel: w1668 -> [w1683 w1692]
                        tunnel: w1671 -> [w1682 w1690]
                        tunnel: [w1681 w1691] -> w1670
                        tunnel: w1669 -> [w1680 w1689]
                        frame "ULx", Default {
                          n531 = call-poly <vilib>:"ULx Write.vi"("task in"=w1687, "auto start"=w1682, "data"=w1683, "timeout"=w1680, "error in"=w1686) -> ("task out"=w1685:refnum<k24>, "number of samples written per channel"=w1681:u32, "error out"=w1684:errorcluster)  [unwired: 8 in]
                        }
                        frame "DAQmx" {
                          n532 = call-poly <vilib>:"DAQmx Write.vi"("task/channels in"=w1695, "auto start"=w1690, "data"=w1692, "timeout"=w1689, "error in"=w1696) -> ("task out"=w1694:refnum<k21>, "number of samples written per channel"=w1691:u32, "error out"=w1693:errorcluster)  [unwired: 8 in]
                        }
                      }
                      "data 7" <- w1668
                      "DblArray" <- w1668
                    }
                    frame "nCnS1DWfm" {
                      n533 = case shown="\"ULx\", Default" w1701 {
                        tunnel: [w1714 w1717] -> w1706
                        tunnel: [w1713 w1722] -> w1705
                        tunnel: w1704 -> [w1708 w1724]
                        tunnel: w1703 -> [w1716 w1717]
                        tunnel: w1702 -> [w1715 w1725]
                        tunnel: [w1708 w1723] -> w1707
                        tunnel: w1697 -> [w1712 w1721]
                        tunnel: w1700 -> [w1711 w1720]
                        tunnel: [w1710 w1719] -> w1699
                        tunnel: w1698 -> [w1709 w1718]
                        frame "ULx", Default {
                          n534 = call-poly <vilib>:"ULx Write.vi"("task in"=w1716, "auto start"=w1711, "data"=w1712, "timeout"=w1709, "error in"=w1715) -> ("task out"=w1714:refnum<k24>, "number of samples written per channel"=w1710:u32, "error out"=w1713:errorcluster)  [unwired: 8 in]
                        }
                        frame "DAQmx" {
                          n535 = call-poly <vilib>:"DAQmx Write.vi"("task/channels in"=w1724, "auto start"=w1720, "data"=w1721, "timeout"=w1718, "error in"=w1725) -> ("task out"=w1723:refnum<k21>, "number of samples written per channel"=w1719:u32, "error out"=w1722:errorcluster)  [unwired: 8 in]
                        }
                      }
                      "data 8" <- w1697
                    }
                    frame "2DI16" {
                      n536 = case shown="\"ULx\", Default" w1729 {
                        tunnel: [w1738 w1747] -> w1730
                        tunnel: [w1737 w1739] -> w1731
                        tunnel: w1733 -> [w1738 w1745]
                        tunnel: w1734 -> [w1737 w1739]
                        tunnel: [w1736 w1746] -> w1732
                        tunnel: w1735 -> [w1736 w1744]
                        tunnel: w1728 -> [_ w1742]
                        tunnel: [_ w1741] -> w1727
                        tunnel: w1726 -> [_ w1740]
                        frame "ULx", Default {
                        }
                        frame "DAQmx" {
                          n537 = call-poly <vilib>:"DAQmx Write.vi"("task/channels in"=w1744, "auto start"=w1742, "data"="data 9", "timeout"=w1740, "error in"=w1745) -> ("task out"=w1746:refnum<k21>, "number of samples written per channel"=w1741:u32, "error out"=w1747:errorcluster)  [unwired: 8 in]
                        }
                      }
                    }
                    frame "2DI32" {
                      n538 = case shown="\"ULx\", Default" w1751 {
                        tunnel: [w1759 w1768] -> w1754
                        tunnel: [w1760 w1761] -> w1753
                        tunnel: w1757 -> [w1759 w1769]
                        tunnel: w1756 -> [w1760 w1761]
                        tunnel: [w1758 w1766] -> w1752
                        tunnel: w1755 -> [w1758 w1767]
                        tunnel: w1750 -> [_ w1764]
                        tunnel: w1749 -> [_ w1763]
                        tunnel: [_ w1762] -> w1748
                        frame "ULx", Default {
                        }
                        frame "DAQmx" {
                          n539 = call-poly <vilib>:"DAQmx Write.vi"("task/channels in"=w1767, "auto start"=w1764, "data"="data 10", "timeout"=w1763, "error in"=w1769) -> ("task out"=w1766:refnum<k21>, "number of samples written per channel"=w1762:u32, "error out"=w1768:errorcluster)  [unwired: 8 in]
                        }
                      }
                    }
                    frame "2DU16" {
                      n540 = case shown="\"ULx\", Default" w1773 {
                        tunnel: [w1781 w1790] -> w1776
                        tunnel: [w1782 w1783] -> w1775
                        tunnel: w1779 -> [w1781 w1791]
                        tunnel: w1778 -> [w1782 w1783]
                        tunnel: [w1780 w1788] -> w1774
                        tunnel: w1777 -> [w1780 w1789]
                        tunnel: w1772 -> [_ w1786]
                        tunnel: w1771 -> [_ w1785]
                        tunnel: [_ w1784] -> w1770
                        frame "ULx", Default {
                        }
                        frame "DAQmx" {
                          n541 = call-poly <vilib>:"DAQmx Write.vi"("task/channels in"=w1789, "auto start"=w1786, "data"="data 11", "timeout"=w1785, "error in"=w1791) -> ("task out"=w1788:refnum<k21>, "number of samples written per channel"=w1784:u32, "error out"=w1790:errorcluster)  [unwired: 8 in]
                        }
                      }
                    }
                  }
                }
                frame "Digital" {
                  n542 = case shown="\"Single Channel\"" "nOrsDChan" {
                    tunnel: w1804 -> [w1815 w2118]
                    tunnel: w1803 -> [w1814 w2119]
                    tunnel: w1802 -> [w1813 w2120]
                    tunnel: w1801 -> [w1812 w2117]
                    tunnel: [w1810 w2116] -> w1799
                    tunnel: [w1809 w2115] -> w1798
                    tunnel: [w1808 w2114] -> w1797
                    tunnel: w1796 -> [w1806 w2113]
                    tunnel: w1795 -> [w1807 w2112]
                    tunnel: [w1805 w2111] -> w1794
                    tunnel: w1793 -> [_ w2109]
                    tunnel: w1792 -> [_ w2108]
                    frame "Multi-Channel", Default {
                      n543 = case shown="\"nCsS2D\"" "nDWrite" {
                        tunnel: [w1825 w1855 w1883 w1913 w1941 w1970 w1999 w2029 w2057 w2087] -> w1808
                        tunnel: [w1826 w1854 w1884 w1912 w1942 w1971 w2000 w2028 w2058 w2086] -> w1809
                        tunnel: w1812 -> [w1824 w1852 w1882 w1911 w1939 w1969 w1998 w2027 w2056 w2085]
                        tunnel: w1814 -> [w1822 w1853 w1880 w1909 w1938 w1967 w1996 w2025 w2055 w2084]
                        tunnel: w1813 -> [w1823 w1850 w1878 w1907 w1936 w1966 w1995 w2023 w2052 w2083]
                        tunnel: w1815 -> [w1821 w1851 w1881 w1910 w1940 w1968 w1997 w2026 w2054 w2082]
                        tunnel: [w1820 w1849 w1879 w1908 w1937 w1965 w1994 w2024 w2053 w2081] -> w1810
                        tunnel: w1807 -> [w1818 w1847 w1876 w1905 w1934 w1963 w1992 w2021 w2050 w2079]
                        tunnel: w1806 -> [w1817 w1846 w1875 w1904 w1933 w1961 w1991 w2020 w2049 w2078]
                        tunnel: [w1816 w1845 w1874 w1903 w1932 w1962 w1990 w2019 w2048 w2077] -> w1805
                        frame "nCsSBool", Default {
                          n544 = case shown="\"ULx\", Default" w1824 {
                            tunnel: [w1832 w1836] -> w1826
                            tunnel: [w1833 w1841] -> w1825
                            tunnel: w1823 -> [w1827 w1844]
                            tunnel: w1822 -> [w1835 w1836]
                            tunnel: w1821 -> [w1834 w1842]
                            tunnel: [w1827 w1843] -> w1820
                            tunnel: "data 12" -> [w1831 w1840]
                            tunnel: w1818 -> [w1830 w1839]
                            tunnel: w1817 -> [w1829 w1838]
                            tunnel: [w1828 w1837] -> w1816
                            frame "ULx", Default {
                              n545 = call-poly <vilib>:"ULx Write.vi"("task in"=w1835, "auto start"=w1829, "data"=w1831, "timeout"=w1830, "error in"=w1834) -> ("task out"=w1832:refnum<k24>, "number of samples written per channel"=w1828:u32, "error out"=w1833:errorcluster)  [unwired: 8 in]
                            }
                            frame "DAQmx" {
                              n546 = call-poly <vilib>:"DAQmx Write.vi"("task/channels in"=w1844, "auto start"=w1838, "data"=w1840, "timeout"=w1839, "error in"=w1842) -> ("task out"=w1843:refnum<k21>, "number of samples written per channel"=w1837:u32, "error out"=w1841:errorcluster)  [unwired: 8 in]
                            }
                          }
                        }
                        frame "nCsS2D" {
                          n547 = case shown="\"ULx\", Default" w1852 {
                            tunnel: [w1862 w1870] -> w1855
                            tunnel: [w1861 w1865] -> w1854
                            tunnel: w1853 -> [w1864 w1865]
                            tunnel: w1851 -> [w1863 w1872]
